vi "EnableCurrentOutput.vi"(2 "error out 2":errorcluster, 3 "reference out 2":refnum<visa-resource-name>) -> (0 "error out":errorcluster, 1 "reference out":refnum<visa-resource-name>)   [LabVIEW 2009]
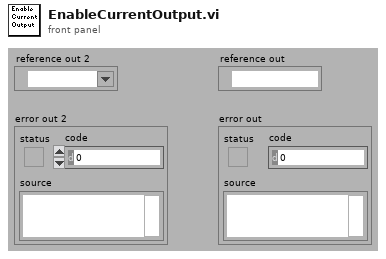
[diagram p1: front panel]
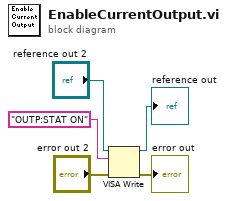
[diagram p0: block diagram]
diagram:
  n1 = VISA Write(VISA resource name="reference out 2", write buffer="OUTP:STAT ON", error in (no error)="error out 2") -> (VISA resource name out=→"reference out":refnum<visa-resource-name>, error out=→"error out":errorcluster)  [unwired: 1 out]
